vi "Initialize Acyclic Frames.vi"(6 "bus controller":T2, 8 "error in":errorcluster, 9 "next available buffer id":u16, 10 "bc address to \nbuffer id map":T1, 11 "module handle":u32) -> (0 "error out":errorcluster, 1 "next available buffer id out":u16, 2 "bc address to buffer id map out":T1, 3 "module handle out":u32)   [LabVIEW 2020, in "AIM MIL-STD-1553 Engine.lvlib" / "Implementation.lvlib" / "Shared Resources.lvclass"]
uses:
  Shared Resources.lvclass
  BC Subaddress to Buffer ID Map.ctl
  Custom Device/Bus Controller Configuration.ctl
  Custom Device/Major Frame Configuration.ctl
  Custom Device/Minor Frame Configuration.ctl
  Custom Device/Acyclic Frame Configuration.ctl
  Custom Device/Message Configuration.ctl
  <instrlib>/_AIM MIL-STD-1553/AIM Controls/1553 Transfer Descriptor.ctl
  <vilib>/Utility/miscctls.llb/LVMapReplaceAction.ctl
  Hardware API/AIM MIL-STD-1553 Hardware API.lvlib
  Custom Device/Custom Device.lvlib
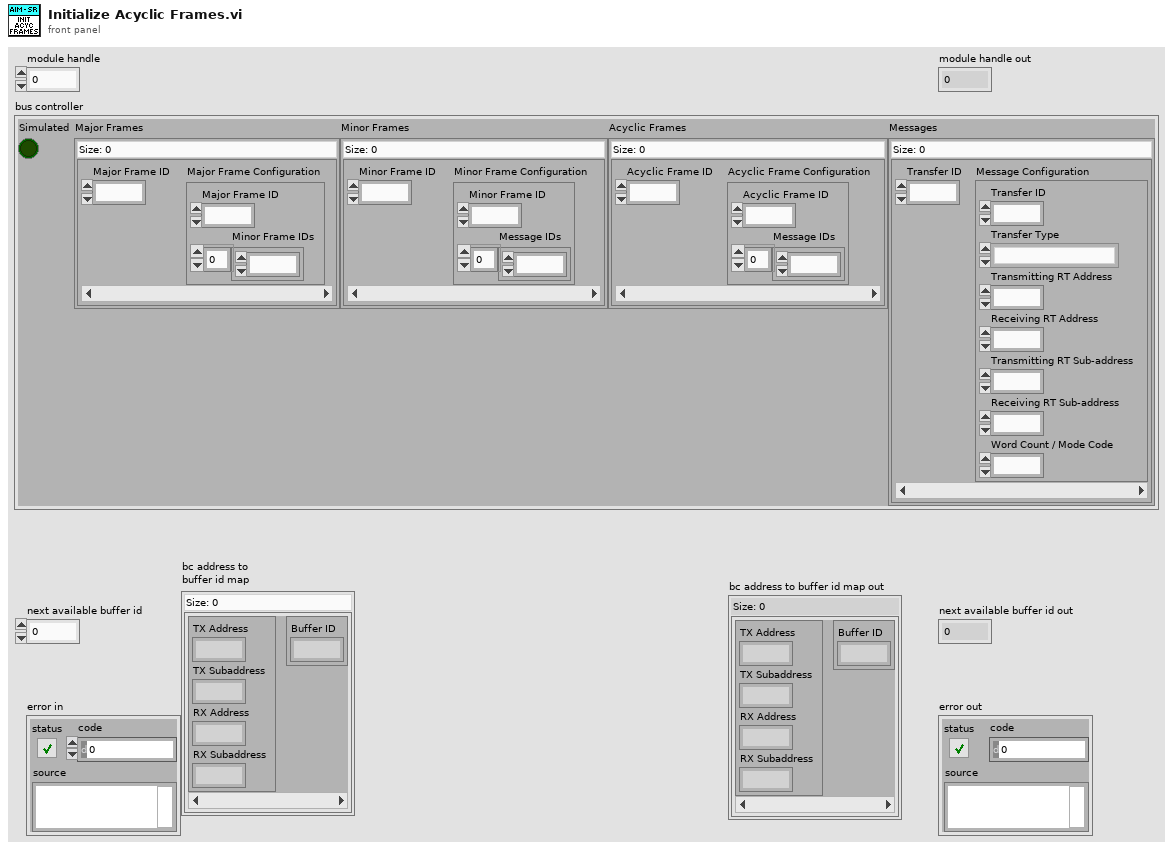
[diagram p1: front panel]
types:
  T1 = typedef "AIM MIL-STD-1553 Engine.lvlib/Implementation.lvlib/Shared Resources.lvclass/BC Subaddress to Buffer ID Map.ctl" = map{cluster{"TX Address":u8, "TX Subaddress":u8, "RX Address":u8, "RX Subaddress":u8}, cluster{"Buffer ID":u16}}
  T2 = typedef "AIM MIL-STD-1553 Engine.lvlib/Custom Device.lvlib/Bus Controller Configuration.ctl" = cluster{"Simulated":bool, "Major Frames":map{u8, T3}, "Minor Frames":map{u8, T4}, "Acyclic Frames":map{u8, T5}, "Messages":map{u16, T6}}
  T3 = typedef "AIM MIL-STD-1553 Engine.lvlib/Custom Device.lvlib/Major Frame Configuration.ctl" = cluster{"Major Frame ID":u8, "Minor Frame IDs":u8[]}
  T4 = typedef "AIM MIL-STD-1553 Engine.lvlib/Custom Device.lvlib/Minor Frame Configuration.ctl" = cluster{"Minor Frame ID":u8, "Message IDs":u16[]}
  T5 = typedef "AIM MIL-STD-1553 Engine.lvlib/Custom Device.lvlib/Acyclic Frame Configuration.ctl" = cluster{"Acyclic Frame ID":u8, "Message IDs":u16[]}
  T6 = typedef "AIM MIL-STD-1553 Engine.lvlib/Custom Device.lvlib/Message Configuration.ctl" = cluster{"Transfer ID":u16, "Transfer Type":enum16{"BC to RT transfer", "RT to BC transfer", "RT to RT transfer"}, "Transmitting RT Address":u8, "Receiving RT Address":u8, "Transmitting RT Sub-address":u8, "Receiving RT Sub-address":u8, "Word Count / Mode Code":u8}
  T7 = typedef "1553 Transfer Descriptor.ctl" = cluster{"Transfer ID":u16, "Buffer Header ID":u16, "Transfer Type":enum16{"BC to RT transfer", "RT to BC transfer", "RT to RT transfer"}, "Bus":enum16{"primary", "secondary"}, "Transmitting RT Address":u8, "Receiving RT Address":u8, "Transmitting RT Sub-address":u8, "Receiving RT Sub-address":u8, "Word Count / Mode Code":u8, "Interrupt Control":enum16{"none", "on end of transfer", "on transfer error", "on status word exception"}, "Halt Control":enum16{"none", "on transfer error", "on status word exception", "on both", "on any interrupt"}, "Retry Control":enum16{"disable", "enable", "keep bus at next transmit", "alternate bus on next transmit"}, "Expected Response":enum16{"automatic", "no status word 1", "no status word 2"}, "Gap Mode":enum16{"delay", "standard", "fast"}, "Transfer Wait Time":u16}
  T8 = typedef "LVMapReplaceAction.ctl" = enum32{"Modify Entry only if found", "Add or Modify Entry", "Delete Entry"}
  T9 = enum16{"BC to RT transfer", "RT to BC transfer", "RT to RT transfer"}
  T10 = cluster{"Transmitting RT Address":u8, "Transmitting RT Sub-address":u8, "Receiving RT Address":u8, "Receiving RT Sub-address":u8}
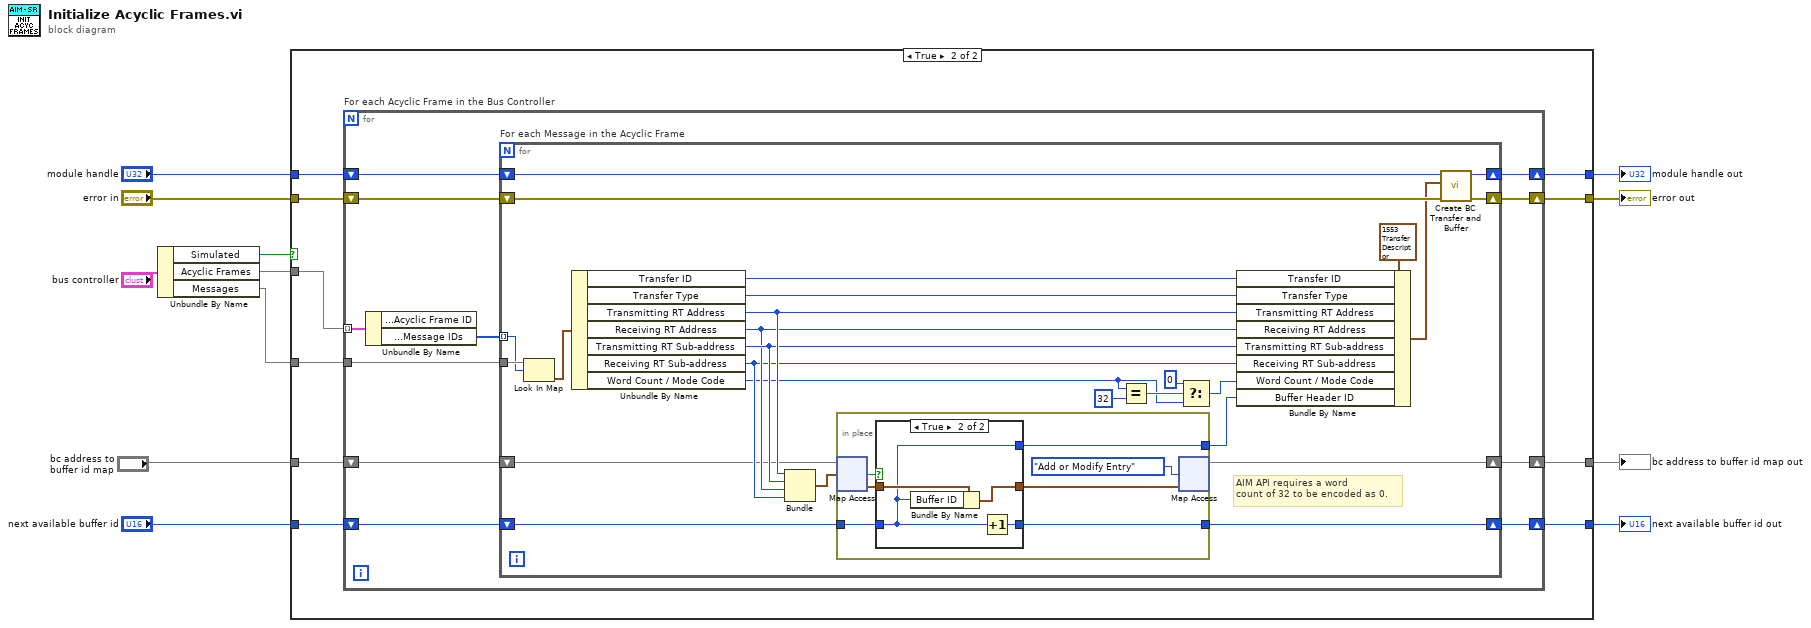
[diagram p0: block diagram]
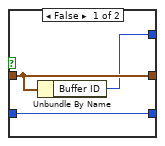
[diagram p3: hidden frame]
diagram:
  n1 = Unbundle By Name("bus controller") -> ("Simulated"=w7:bool, "Acyclic Frames"=w2:map{u8, T5}, "Messages"=w3:map{u16, T6})
  n2 = case shown="True" w7 {
    tunnel: w2 -> [_ w18]
    tunnel: w3 -> [_ w25]
    tunnel: "module handle" -> [w14 w16]
    tunnel: "error in" -> [w13 w17]
    tunnel: "next available buffer id" -> [w15 w24]
    tunnel: [w14 w23] -> w5
    tunnel: [w13 w22] -> w6
    tunnel: [w15 w21] -> w11
    tunnel: [_ w20] -> w12
    tunnel: "bc address to \nbuffer id map" -> [_ w19]
    frame False {
    }
    frame True {
      n3 = for "For each Acyclic Frame in the Bus Controller" {
        tunnel: w18 -> [w26] mode=indexing
        tunnel: w25 -> [w35]
        shift-right: [w32] -> w22
        shift-left: w17 -> [w33]
        shift-right: [w31] -> w23
        shift-left: w16 -> [w34]
        shift-right: [w29] -> w21
        shift-left: w24 -> [w30]
        shift-right: [w27] -> w20
        shift-left: w19 -> [w28]
        n4 = Unbundle By Name(w26) -> ("Acyclic Frame Configuration.Message IDs"=w36:u16[])  [unwired: 1 out]
        n5 = for "For each Message in the Acyclic Frame" {
          tunnel: w36 -> [w60] mode=indexing
          tunnel: w35 -> [w61]
          shift-right: [w56] -> w32
          shift-left: w33 -> [w57]
          shift-right: [w55] -> w31
          shift-left: w34 -> [w58]
          shift-right: [w52] -> w29
          shift-left: w30 -> [w53]
          shift-right: [w45] -> w27
          shift-left: w28 -> [w46]
          # "AIM API requires a word \ncount of 32 to be encoded as 0."
          n6 = Look In Map(map=w61, key=w60) -> (value=w59:T6)  [unwired: 1 in, 1 out]
          n7 = Unbundle By Name(w59) -> ("Transfer ID"=w54:u16, "Transfer Type"=w51:T9, "Transmitting RT Address"=w50:u8, "Receiving RT Address"=w48:u8, "Transmitting RT Sub-address"=w49:u8, "Receiving RT Sub-address"=w47:u8, "Word Count / Mode Code"=w38:u8)
          n8 = Bundle("Transmitting RT Address"=w50, "Transmitting RT Sub-address"=w49, "Receiving RT Address"=w48, "Receiving RT Sub-address"=w47) -> (w44:T10)  [unwired: 1 in]
          n9 = in-place {
            in-place-border: w53 -> [w68]
            in-place-border: [w66] -> w52
            in-place-border: [w63] -> w43
            n10 = in-place-map #1(w46, w44) -> (w65:cluster{"Buffer ID":u16}, w69:bool)  [unwired: 1 in]
            n11 = case shown="True" w69 {
              tunnel: w68 -> [w72 w73]
              tunnel: [w71 w74] -> w64
              tunnel: [w72 w76] -> w66
              tunnel: w65 -> [w71 w75]
              tunnel: [w70 w73] -> w63
              frame False {
                n12 = Unbundle By Name(w71) -> ("Buffer ID"=w70:u16)
              }
              frame True {
                n13 = Bundle By Name(cluster=w75, "Buffer ID"=w73) -> (w74:cluster{"Buffer ID":u16})
                n14 = Increment(x=w73) -> (x+1=w76:u16)
              }
            }
            n15 = in-place-map #1(w64, LVMapReplaceAction."Add or Modify Entry" ("action")) -> (w45:T1)  [unwired: 2 out]
          }
          n16 = Equal?(x=w38, y=u8 32) -> (x = y?=w41:bool)
          n17 = Select(t=u8 0, s=w41, f=w38) -> (s? t:f=w39:u8)
          n18 = Bundle By Name(cluster=T7 {"Transfer ID"=0, "Buffer Header ID"=0, "Transfer Type"=enum."BC to RT transfer", "Bus"=enum."primary", "Transmitting RT Address"=0, "Receiving RT Address"=0, "Transmitting RT Sub-address"=0, "Receiving RT Sub-address"=0, "Word Count / Mode Code"=0, "Interrupt Control"=enum."none", "Halt Control"=enum."none", "Retry Control"=enum."disable", "Expected Response"=enum."automatic", "Gap Mode"=enum."delay", "Transfer Wait Time"=0} ("BC Transfer Descriptor"), "Transfer ID"=w54, "Transfer Type"=w51, "Transmitting RT Address"=w50, "Receiving RT Address"=w48, "Transmitting RT Sub-address"=w49, "Receiving RT Sub-address"=w47, "Word Count / Mode Code"=w39, "Buffer Header ID"=w43) -> (w37:T7)
          n19 = call "Create BC Transfer and Buffer.vi"("error in"=w57, "bc transfer descriptor"=w37, "module handle"=w58) -> ("error out"=w56:errorcluster, "module handle out"=w55:u32)  [unwired: 6 in, 1 out]
        }
      }
    }
  }
  "bc address to buffer id map out" <- w12
  "next available buffer id out" <- w11
  "error out" <- w6
  "module handle out" <- w5
